vi "OWC.vi"() -> ()   [LabVIEW 2020]
uses:
  Private/Type Defs/HSB.ctl
  512cd6d3-8cdb-454e-9b2b-47ee723148b5.vi
  145577b0-8988-4740-a407-e11081626666.vi
  Private/Build State URL.vi
  512cd6d3-8cdb-454e-9b2b-47ee723148b5.vi/f10edee5-3db4-4843-a358-6f175c3e5c4d.vi
  Private/Convert HSB.vi
  145577b0-8988-4740-a407-e11081626666.vi/fd3ec008-1d2f-4e71-8ae3-8f5a43173b55.vi
  <vilib>/JDP Science/JSONtext/Variant to JSON Text.vi
  <vilib>/httpClient/PUT.vi
  <vilib>/httpClient/PUTBuffer.vi
  LMH-Hue.lvlib
panel:
  out "<JSON>":string
  out "Response":string
  in  "HSB":T1={"Hue"=0, "Saturation"=255, "Brightness"=255}
  in  "Stop Button":bool
  in  "Hostname / IP":string="192.168.1.3"
  in  "Username":string="n2E5i0EwzIpdamkjJWehfzOrC8RPhy6IB12A83ts"
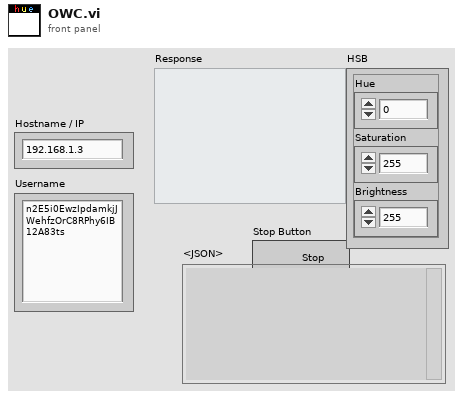
[diagram p1: front panel]
types:
  T1 = typedef "LMH-Hue.lvlib/HSB.ctl" = cluster{"Hue":u16, "Saturation":u8, "Brightness":u8}
  T2 = typedef "LMH-Hue.lvlib/Hue Ref.ctl" = cluster{"HTTP Session":T3, "Base URL":string, "Map":map{i32, T4}}
  T3 = typedef "LabVIEWHTTPClient.lvlib/ClientHandle.ctl" = refnum<k1>
  T4 = typedef "LMH-Hue.lvlib/Light Data.ctl" = cluster{"Name":string, "On?":bool, "Reachable?":bool, "Color?":bool}
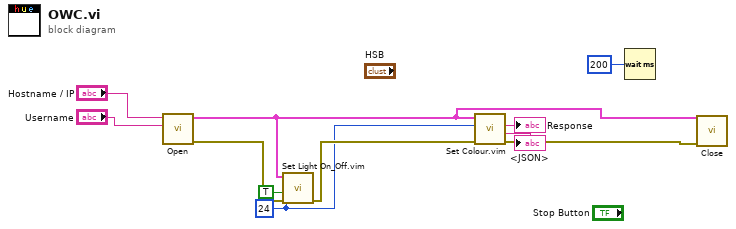
[diagram p0: block diagram]
diagram:
  w2 = u8 24 ("ID")
  n1 = call "Open.vi"("Username"="Username", "Hostname / IP"="Hostname / IP") -> ("Error Out"=w6:errorcluster, "Hue Config"=w9:T2)  [unwired: 8 in]
  n2 = call "Set Light On_Off.vim"("error in"=w6, "Light Control"=TRUE, "ID"=w2, "Hue Config"=w9) -> ("error out"=w5:errorcluster)  [unwired: 6 in, 1 out]
  n3 = call "Set Colour.vim"("error in"=w5, "ID"=w2, "Hue Config"=w9) -> ("error out"=w8:errorcluster, "<JSON>"=→"<JSON>":string, "Response"=→"Response":string)  [unwired: 6 in]
  n4 = Wait (ms)(milliseconds to wait=u32 200 ("Delay")) -> ()  [unwired: 1 out]
  n5 = call "Close.vi"("Error In"=w8, "Hue Config"=w9) -> ()  [unwired: 9 in, 1 out]
